vi "TemplateModule.Start.vi"(5 "Autoshutdown? (T)":bool=TRUE, 8 "error in (no error)":errorcluster, 11 "TemplateModule in":refnum<class "TemplateModule.lvclass">) -> (0 "error out":errorcluster, 1 "StartupHandshake out":refnum<class "RQMHStartup.lvclass">, 2 "_TemplateModule":cluster{"Broadcasts":T1, "Broadcasts":T2}, 3 "TemplateModule out":refnum<class "TemplateModule.lvclass">)   [LabVIEW 2024, in "TemplateModule.lvclass"]
uses:
  TemplateModule.lvclass
  C:/Github/JQMH/JQMHCore/Module/RQMHModule.lvclass
  JQMHCore/Module/StandardBroadcasts.ctl
  JQMHCore/Shared/Died.ctl
  JQMHCore/Module/Started.ctl
  Broadcast Events--cluster.ctl
  Stopped.ctl
  JamesBroad.ctl
  JQMHCore/Module/RQMHModule.lvclass
  JQMHCore/JQMHStartup/RQMHStartup.lvclass
  TemplateModule.lvclass/TemplateModule.ctl
  JQMHCore/Shared/RQMHShared.lvlib
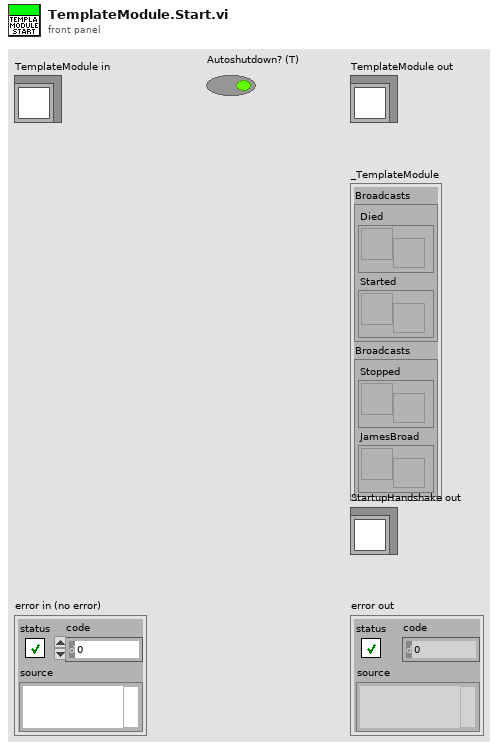
[diagram p1: front panel]
types:
  T1 = typedef "RQMHModule.lvclass/StandardBroadcasts.ctl" = cluster{"Died":refnum<user-event>, "Started":refnum<user-event>}
  T2 = typedef "TemplateModule.lvclass/Broadcast Events--cluster.ctl" = cluster{"Stopped":refnum<user-event>, "JamesBroad":refnum<user-event>}
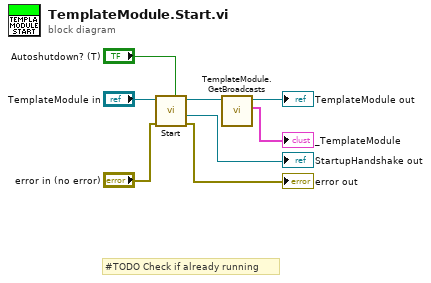
[diagram p0: block diagram]
diagram:
  # "#TODO Check if already running"
  n1 = call "Start.vi"("Autoshutdown? (T)"="Autoshutdown? (T)", "error in (no error)"="error in (no error)", "JQMHCore in"="TemplateModule in") -> ("error out"=→"error out":errorcluster, "StartupHandshake out"=→"StartupHandshake out":refnum<class "RQMHStartup.lvclass">, "JQMHCore out"=w4:refnum<class "TemplateModule.lvclass">)  [unwired: 6 in]
  n2 = call "TemplateModule.GetBroadcasts.vi"("TemplateModule in"=w4) -> ("TemplateModule"=→"_TemplateModule":cluster{"Broadcasts":T1, "Broadcasts":T2}, "TemplateModule out"=→"TemplateModule out":refnum<class "TemplateModule.lvclass">)  [unwired: 9 in]
